vi "Test Calculate Possible Solutions.vi"() -> ()   [LabVIEW 2025]
uses:
  Controls/Must Contain.ctl
  Controls/Character Position Possible Letters.ctl
  <vilib>/addons/_JKI Toolkits/Caraya/classes/Assert/Assert Equal Value_Variant.vi
  Libraries/WordleSolver/WordleSolver.lvlib
  <vilib>/addons/_JKI Toolkits/Caraya/classes/Test/Test.lvclass
  <vilib>/addons/_JKI Toolkits/Caraya/classes/Assert/Assert.lvclass
panel:
  out "error out":errorcluster
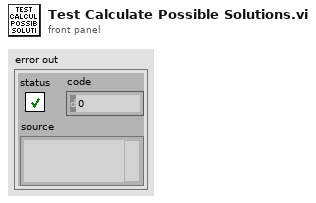
[diagram p1: front panel]
types:
  T1 = typedef "Character Position Possible Letters.ctl" = string[]
  T2 = typedef "Must Contain.ctl" = string
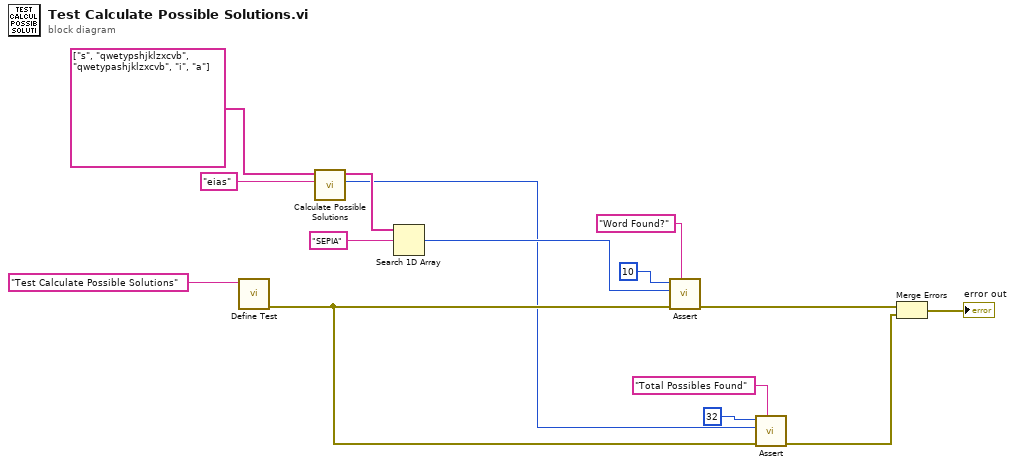
[diagram p0: block diagram]
diagram:
  n1 = call <vilib>:"Define Test.vi"("Label (VI Title)"="Test Calculate Possible Solutions") -> ("error out"=w6:errorcluster)  [unwired: 9 in, 1 out]
  n2 = call "Calculate Possible Solutions.vi"("Must Contain"=T2 "eias", "Character Position Possible Letters"=T1 ["s", "qwetypshjklzxcvb", "qwetypashjklzxcvb", "i", "a"]) -> ("Possible Amount"=w5:i32, "Possibles"=w13:string[])  [unwired: 8 in]
  n3 = Search 1D Array(1D array=w13, element="SEPIA") -> (index of element=w11:i32)  [unwired: 1 in]
  n4 = call-poly <vilib>:"Assert.vi"("Label"="Word Found?", "error in (no error)"=w6, "Actual"=w11, "Expected"=10) -> ("error out"=w8:errorcluster)  [unwired: 6 in, 1 out]
  n5 = call-poly <vilib>:"Assert.vi"("Label"="Total Possibles Found", "error in (no error)"=w6, "Actual"=w5, "Expected"=32) -> ("error out"=w2:errorcluster)  [unwired: 6 in, 1 out]
  n6 = Merge Errors(w8, w2) -> (→"error out":errorcluster)
